vi "Write PRAGMA key Command.vi"(8 "error in (no error)":errorcluster, 10 "PRAGMA key Command":string, 11 "SQLite in":refnum<class "SQLite.lvclass">) -> (0 "error out":errorcluster, 3 "SQLite out":refnum<class "SQLite.lvclass">)   [LabVIEW 2021, in "SQLite.lvclass"]
uses:
  SQLite.lvclass
  SQLite.lvclass/SQLite.ctl
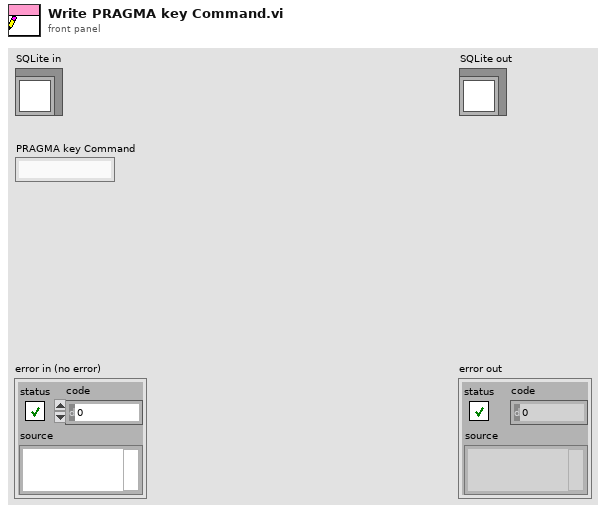
[diagram p1: front panel]
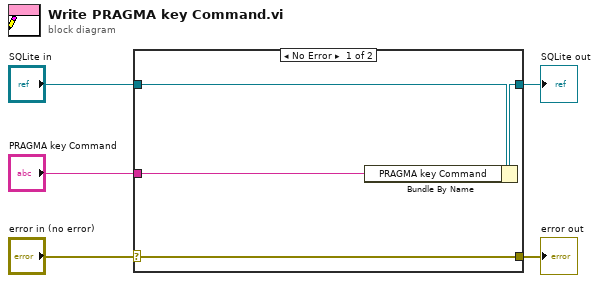
[diagram p0: block diagram]
diagram:
  n1 = case shown="No Error" "error in (no error)" {
    selector: "error in (no error)" -> [w9 w10]
    tunnel: [w9 w10] -> w4
    tunnel: [w7 w11] -> w2
    tunnel: "SQLite in" -> [w8 w11]
    tunnel: "PRAGMA key Command" -> [w6 _]
    frame No Error {
      n2 = Bundle By Name(cluster=w8, "PRAGMA key Command"=w6) -> (w7:refnum<class "SQLite.lvclass">)
    }
    frame Error {
    }
  }
  "error out" <- w4
  "SQLite out" <- w2
